vi "System Exec Build Project.vi"(8 "Error In":errorcluster, 11 "LabVIEW Previous Version In":T1=enum."2015") -> (0 "Error Out":errorcluster, 3 "LabVIEW Previous Version Out":T1=enum."2015")   [LabVIEW 2017]
uses:
  LabVIEW Versions.ctl
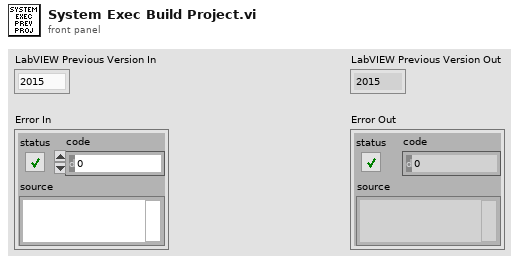
[diagram p1: front panel]
types:
  T1 = typedef "LabVIEW Versions.ctl" = enum16{"2009", "2010", "2011", "2012", "2013", "2014", "2015", "2016", "2017", "2018"}
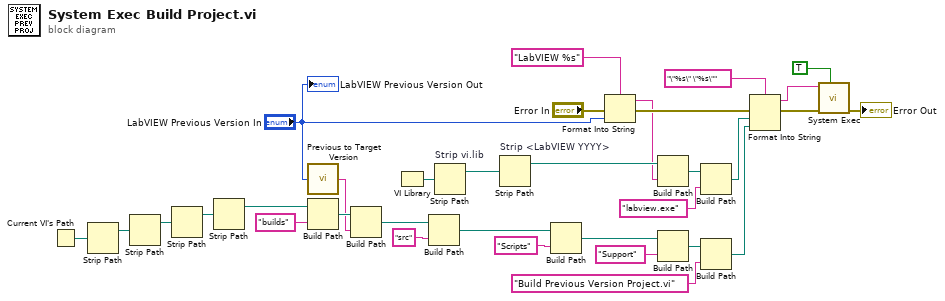
[diagram p0: block diagram]
diagram:
  n1 = Current VI's Path() -> (path=w16:path)
  n2 = Strip Path(path=w16) -> (stripped path=w15:path)  [unwired: 1 out]
  n3 = Strip Path(path=w15) -> (stripped path=w14:path)  [unwired: 1 out]
  n4 = Strip Path(path=w14) -> (stripped path=w13:path)  [unwired: 1 out]
  n5 = Strip Path(path=w13) -> (stripped path=w12:path)  [unwired: 1 out]
  n6 = call "Previous to Target Version.vi"("Previous Version"="LabVIEW Previous Version In") -> ("Target Version"=w9:string)
  n7 = Build Path(base path=w12, name or relative path="builds") -> (appended path=w10:path)
  n8 = Build Path(base path=w10, name or relative path=w9) -> (appended path=w7:path)
  n9 = VI Library() -> (path=w32:path)
  n10 = Build Path(base path=w7, name or relative path="src") -> (appended path=w5:path)
  n11 = Strip Path "Strip vi.lib"(path=w32) -> (stripped path=w31:path)  [unwired: 1 out]
  n12 = Strip Path "Strip <LabVIEW YYYY>"(path=w31) -> (stripped path=w30:path)  [unwired: 1 out]
  n13 = Build Path(base path=w5, name or relative path="Scripts") -> (appended path=w3:path)
  n14 = Format Into String(format string="LabVIEW %s", error in="Error In", "LabVIEW Previous Version In") -> (resulting string=w27:string, error out=w29:errorcluster)  [unwired: 1 in]
  n15 = Build Path(base path=w30, name or relative path=w27) -> (appended path=w26:path)
  n16 = Build Path(base path=w3, name or relative path="Support") -> (appended path=w1:path)
  n17 = Build Path(base path=w26, name or relative path="labview.exe") -> (appended path=w19:path)
  n18 = Build Path(base path=w1, name or relative path="Build Previous Version Project.vi") -> (appended path=w23:path)
  n19 = Format Into String(format string="\"%s\" \"%s\"", error in=w29, w19, w23) -> (resulting string=w18:string, error out=w21:errorcluster)  [unwired: 1 in]
  n20 = call <vilib>:"System Exec.vi"("wait until completion? (T)"=TRUE, "error in (no error)"=w21, "command line"=w18) -> ("error out"=→"Error Out":errorcluster)  [unwired: 5 in, 3 out]
  "LabVIEW Previous Version Out" <- "LabVIEW Previous Version In"
